vi "Trace_UserMsg.vi"(6 "Data":string[](array[string]), 8 "error in (no error)":errorcluster, 9 "Category":string) -> (0 "error out":errorcluster)   [LabVIEW 2018]
uses:
  Tracer.lvclass
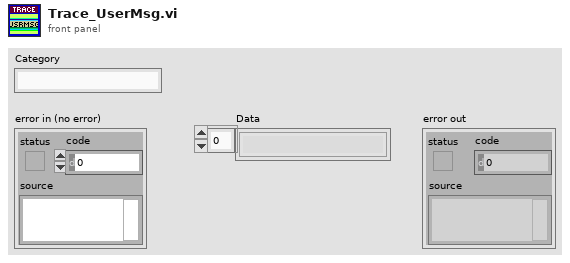
[diagram p1: front panel]
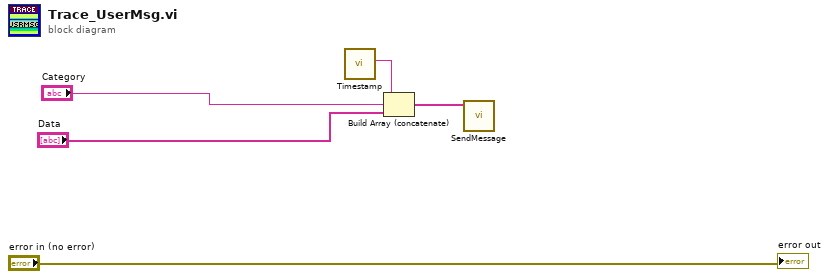
[diagram p0: block diagram]
diagram:
  n1 = call "Timestamp.vi"() -> ("date/time string"=w1:string)  [unwired: 11 in]
  n2 = Build Array (concatenate)(w1, "Category", "Data") -> (w2:string[])
  n3 = call "SendMessage.vi"("Msg"=w2) -> ()  [unwired: 11 in]
  "error out" <- "error in (no error)"
